vi "Async Request Message.vi"(5 "Callback":refnum<class "Callback.lvclass">, 6 "error in (no error)":errorcluster, 7 "Request Message Data":variant, 8 "Request Message":string, 9 "Process In":refnum<class "Process.lvclass">) -> (0 "error out":errorcluster, 3 "Process Out":refnum<class "Process.lvclass">)   [LabVIEW 2020, in "Process.lvclass"]
doc: "Make an asyncronous request to the process. The process should respond to the request made using the Response Message.vi method. When the response is sent from the process, the Callback passed in to this VI is called."
uses:
  Process.lvclass
  C:/git/astemes-triarc-framework/source/Framework/Logging/Logging.lvclass
  Callback/Callback.lvclass
  Message Cluster.ctl
  Process.lvclass/Process.ctl
  Logging/Log Debug.vi
  <vilib>/AdvancedString/1D String Array to Delimited String.vi
  <vilib>/Utility/High Resolution Relative Seconds.vi
  Public/Read Name.vi
  Logging/Logging.lvclass
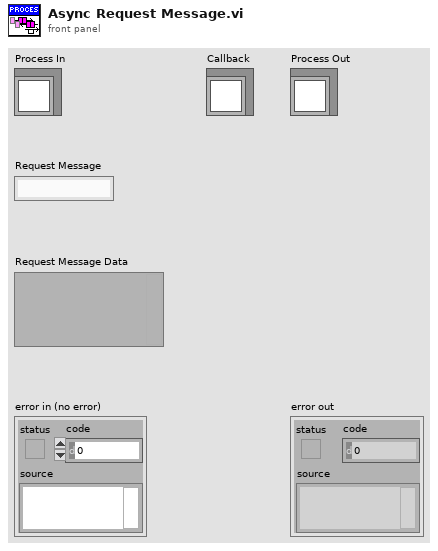
[diagram p1: front panel]
types:
  T1 = typedef "Process.lvclass/Message Cluster.ctl" = cluster{"Message":string, "Message Data":variant, "Request Callback":refnum<class "Callback.lvclass">}
  T2 = enum16{"Send", "Receive", "Request", "Response", "Broadcast"}
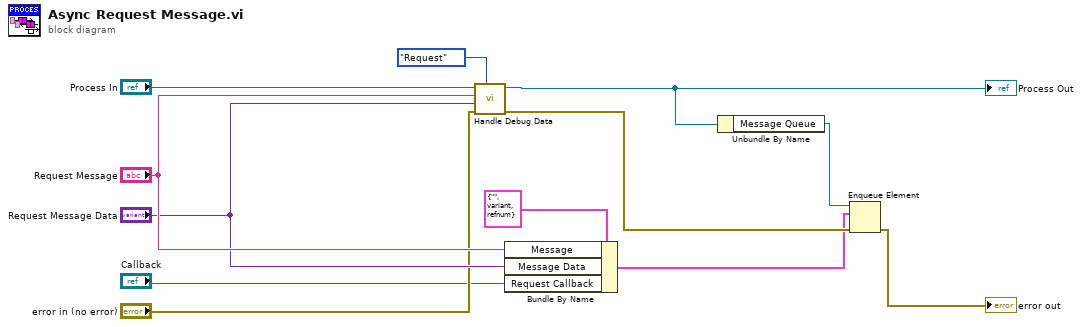
[diagram p0: block diagram]
diagram:
  n1 = call "Handle Debug Data.vi"("Action"=T2."Request", "error in (no error)"="error in (no error)", "Message Data"="Request Message Data", "Message"="Request Message", "Process In"="Process In") -> ("error out"=w7:errorcluster, "Process Out"=w6:refnum<class "Process.lvclass">)  [unwired: 5 in]
  "Process Out" <- w6
  n2 = Bundle By Name(cluster=T1 {"Message"="", "Message Data"=variant, "Request Callback"=refnum} ("Message Cluster"), "Message"="Request Message", "Message Data"="Request Message Data", "Request Callback"="Callback") -> (w3:T1)
  n3 = Unbundle By Name(w6) -> ("Message Queue"=w2:refnum<queue>)
  n4 = Enqueue Element(queue=w2, element=w3, error in (no error)=w7) -> (error out=→"error out":errorcluster)  [unwired: 1 in, 2 out]
